vi "Rod Value Measurement.vi"() -> ()   [LabVIEW 2020]
uses:
  <vilib>/Utility/miscctls.llb/LVAnnotationListTypeDef.ctl
  <vilib>/Utility/miscctls.llb/LVStringsAndValuesArrayTypeDef_U16.ctl
  global/SettingVariable.vi
  <vilib>/Analysis/NI_AALPro.lvlib
panel:
  out "临界段周期":dbl[](array[numeric]) caption="准临界倍增周期 (s)"
  out "临界段反应性拟合值":dbl[](array[numeric]) caption="拟合反应性 (pcm)"
  out "终端反应性均值":dbl[](array[numeric]) caption="实时反应性 (pcm)"
  out "临界段反应性均值":dbl[](array[numeric]) caption="实时反应性 (pcm)"
  out "采样间隔":dbl
  out "开始时间":timestamp
  in  "打开文件":bool
  out "历史波形图":cluster{dbl, dbl, dbl[][]}(graph)
  out "终端段点数":i32 caption="终端段点数："
  out "动态段点数":i32 caption="动态段点数："
  out "左选标时刻":timestamp caption="左选标时刻：" format="%<%.2X %x>T"
  out "临界段点数":i32 caption="临界段点数："
  out "反应性记录表":string[][](table)
  in  "刻棒选择":u16(ring) caption="刻棒选择："
  in  "棒位偏移":dbl(slide) caption="棒位偏移：" min=-0.1 max=0.1 step=0.001 scale=-0.1..0.1 scale format="%#.3g"
  in  "保存表格":bool
  in  "添加记录":bool
  in  "选项卡控件":enum32{"动态段数据", "动态段曲线"}(tab)
  out "棒价值表":string[][](table) caption="动态段"
  in  "另存数据":bool
  out "价值曲线":cluster{dbl[], dbl[]}[](graph) caption="（X和Y数组）多曲线"
  out "提示信息":string="打开文件后，拖动波形图中的游标选取临界段、动态段和终端段数据进行计算。"
  out "文件信息":string
  # "临界段计算结果"
  # "终端段计算结果"
  # "坐标轴与图例"
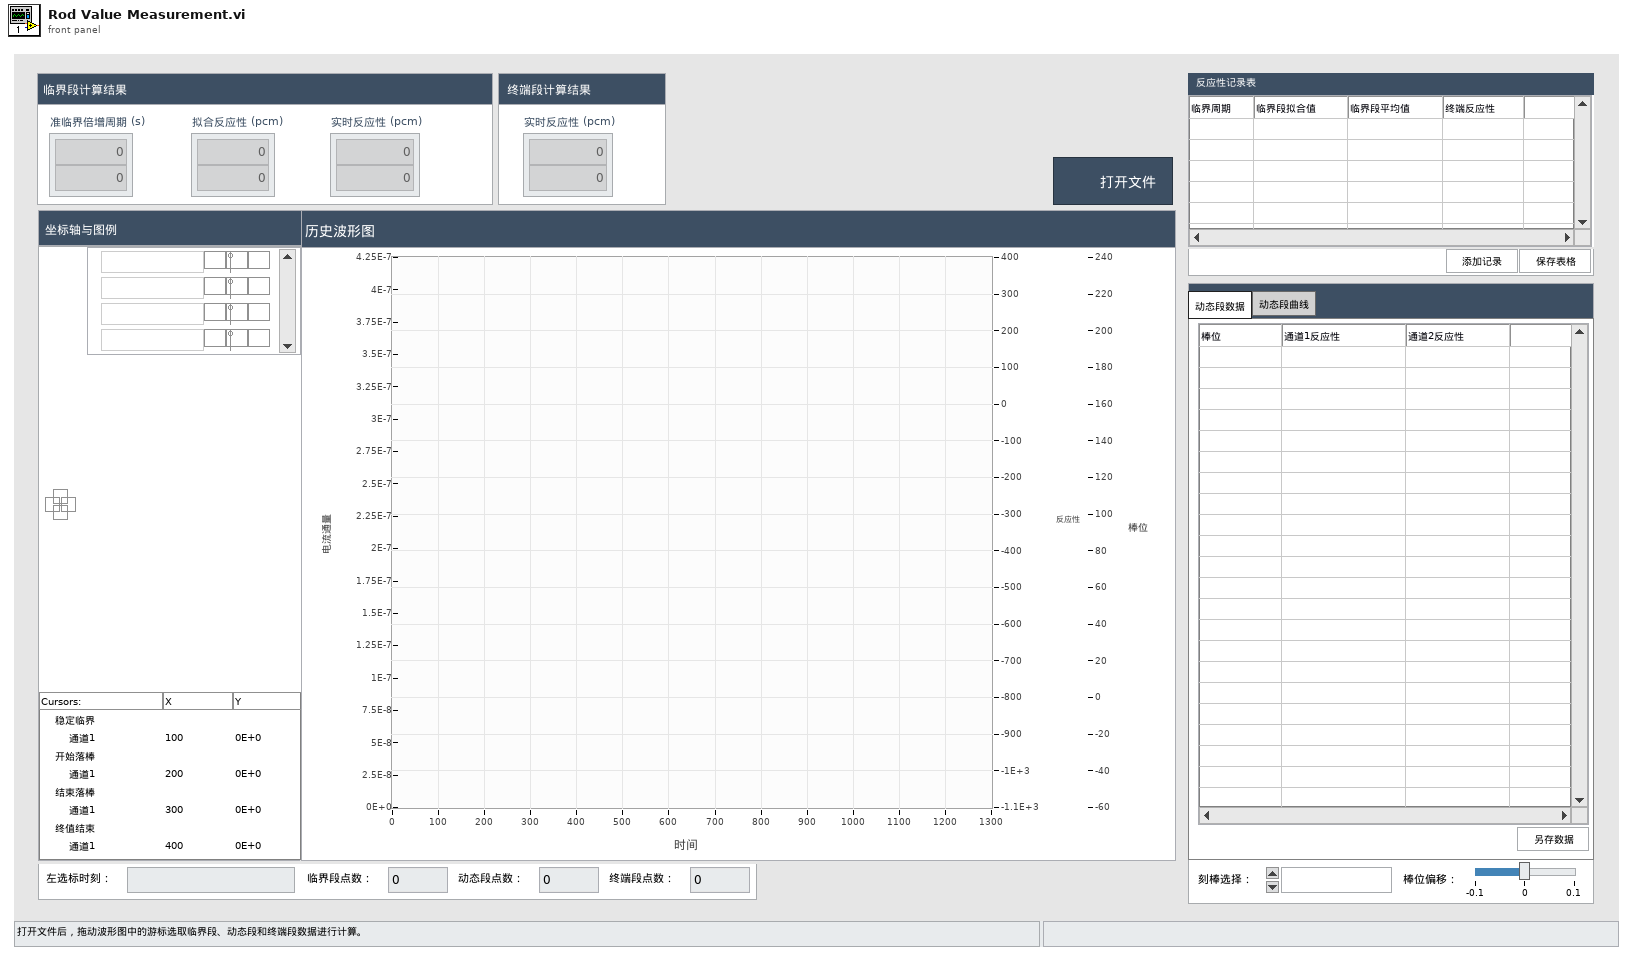
[diagram p1: front panel]
types:
  T1 = typedef "LVAnnotationListTypeDef.ctl" = cluster{"Name":string, "Color":u32, "Style":u8, "Point Style":u8, "Name Visible":bool, "Allow Drag":bool, "Annotation Mode":u32, "Plot":i32, "Index":i32, "Position":cluster{"X":dbl, "Y":dbl}, "X Scale":u32, "Y Scale":u32, "Show Arrow":bool, "Lock Name":bool, "Plot Area":i32, "Label Offset":cluster{"X":dbl, "Y":dbl}}[]
  T2 = typedef "LVStringsAndValuesArrayTypeDef_U16.ctl" = cluster{"String":string, "Value":u16}[]
  T3 = cluster{"Name":string, "Color":u32, "Style":u8, "Point Style":u8, "Name Visible":bool, "Allow Drag":bool, "Annotation Mode":u32, "Plot":i32, "Index":i32, "Position":cluster{"X":dbl, "Y":dbl}, "X Scale":u32, "Y Scale":u32, "Show Arrow":bool, "Lock Name":bool, "Plot Area":i32, "Label Offset":cluster{"X":dbl, "Y":dbl}}
  T4 = cluster{"amp min":dbl, "amp max":dbl, "damping min":dbl, "damping max":dbl, "offset min":dbl, "offset max":dbl}
  T5 = enum16{"open", "replace", "create", "open or create", "replace or create", "replace or create with confirmation"}
  T6 = typedef "LVCursorListTypeDef.ctl" = cluster{"Name":string, "Color":u32, "Style":u8, "Point Style":u8, "Name Visible":bool, "Allow Drag":bool, "Cursor Mode":u32, "Plot":i32, "Index":i32, "Position":cluster{"X":dbl, "Y":dbl}, "X Scale":u32, "Y Scale":u32, "Watch Plots":i32[], "Watch All Plots":bool, "Plot Area":i32, "Label Offset":cluster{"X":dbl, "Y":dbl}}[]
  T7 = cluster{"Name":string, "Color":u32, "Style":u8, "Point Style":u8, "Name Visible":bool, "Allow Drag":bool, "Cursor Mode":u32, "Plot":i32, "Index":i32, "Position":cluster{"X":dbl, "Y":dbl}, "X Scale":u32, "Y Scale":u32, "Watch Plots":i32[], "Watch All Plots":bool, "Plot Area":i32, "Label Offset":cluster{"X":dbl, "Y":dbl}}
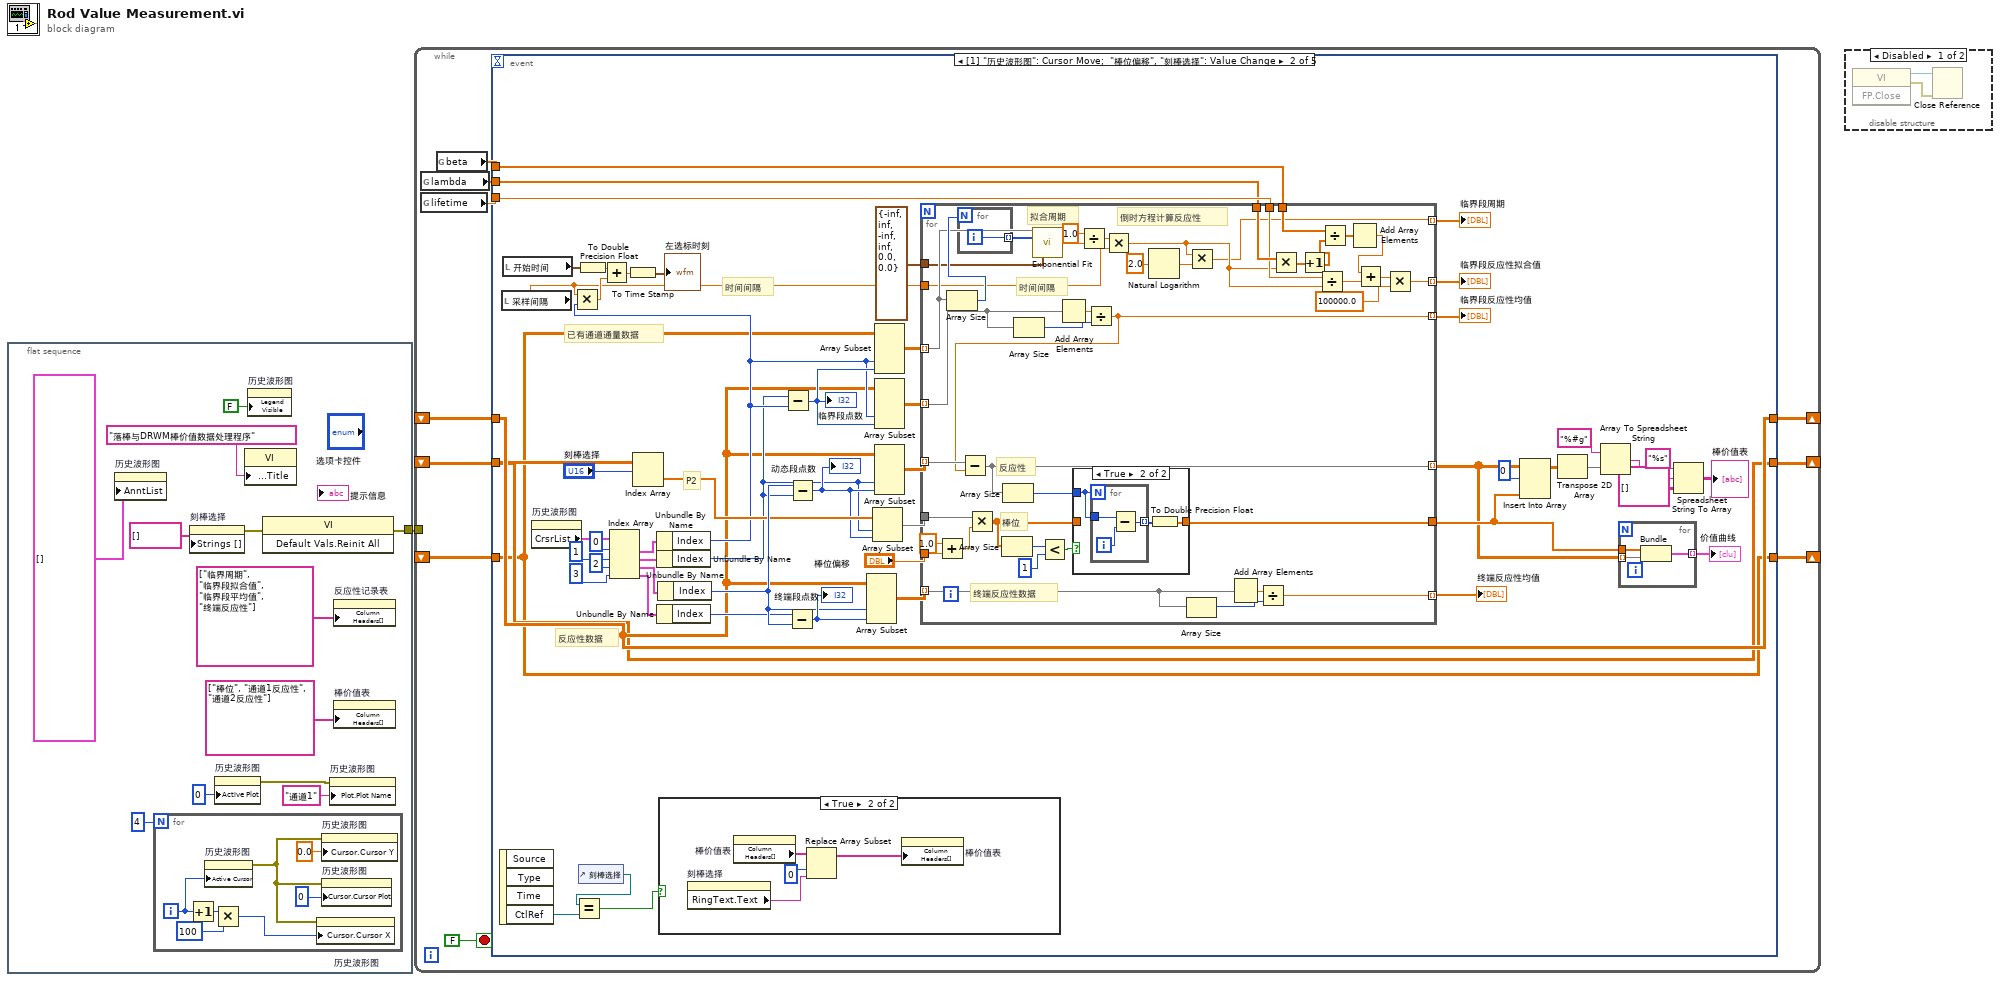
[diagram p0: block diagram]
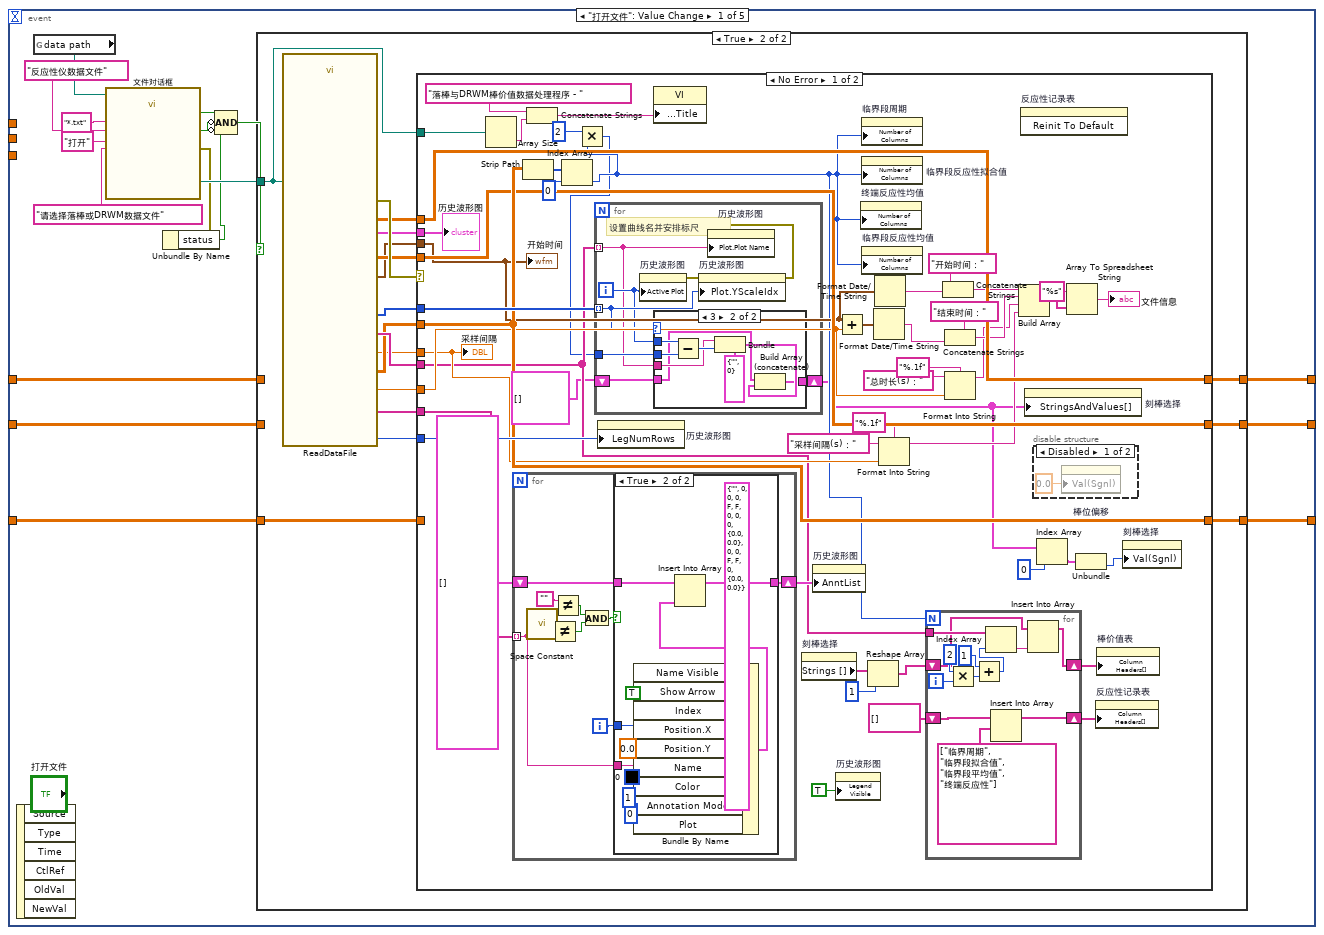
[diagram p2: hidden frame]
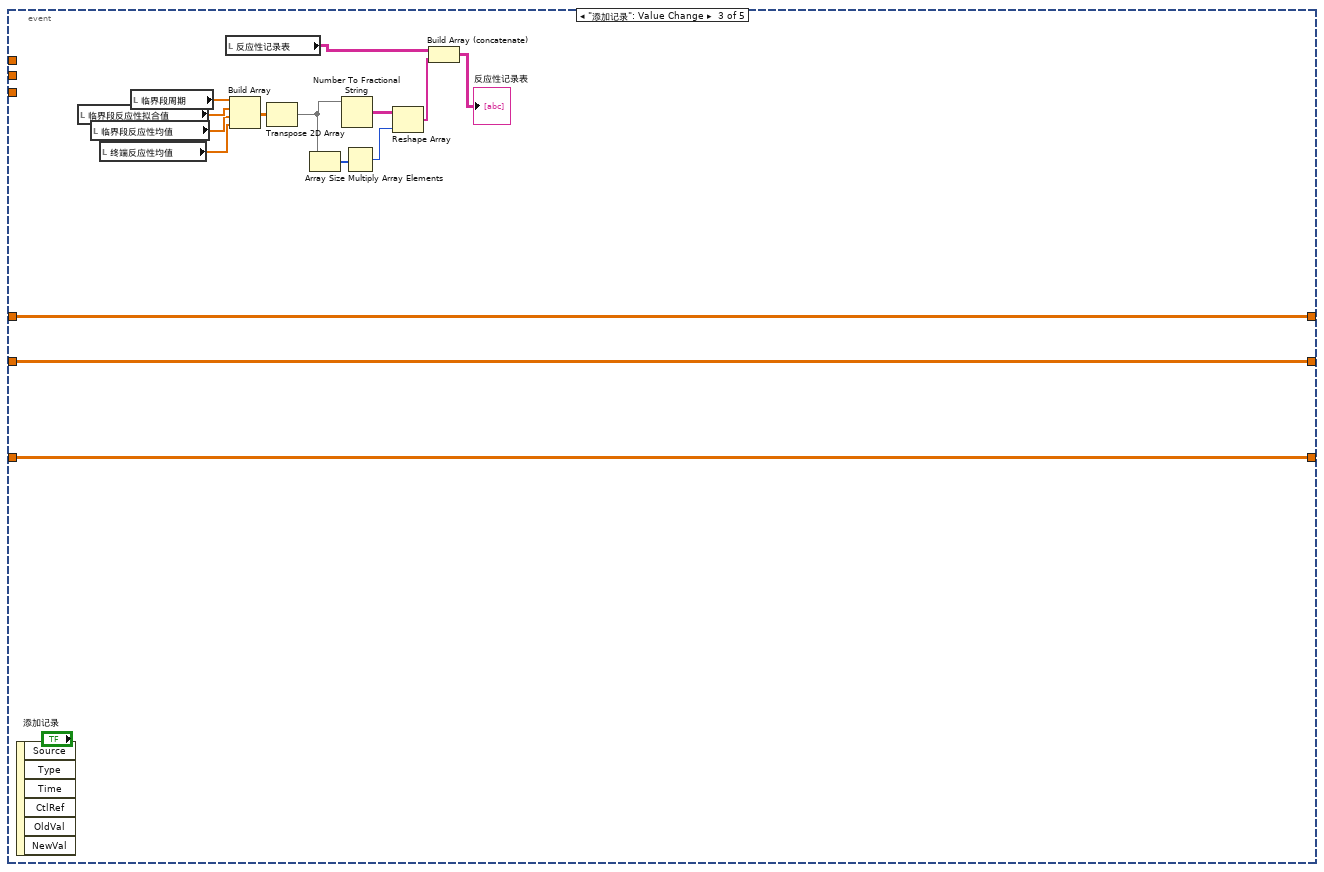
[diagram p10: hidden frame]
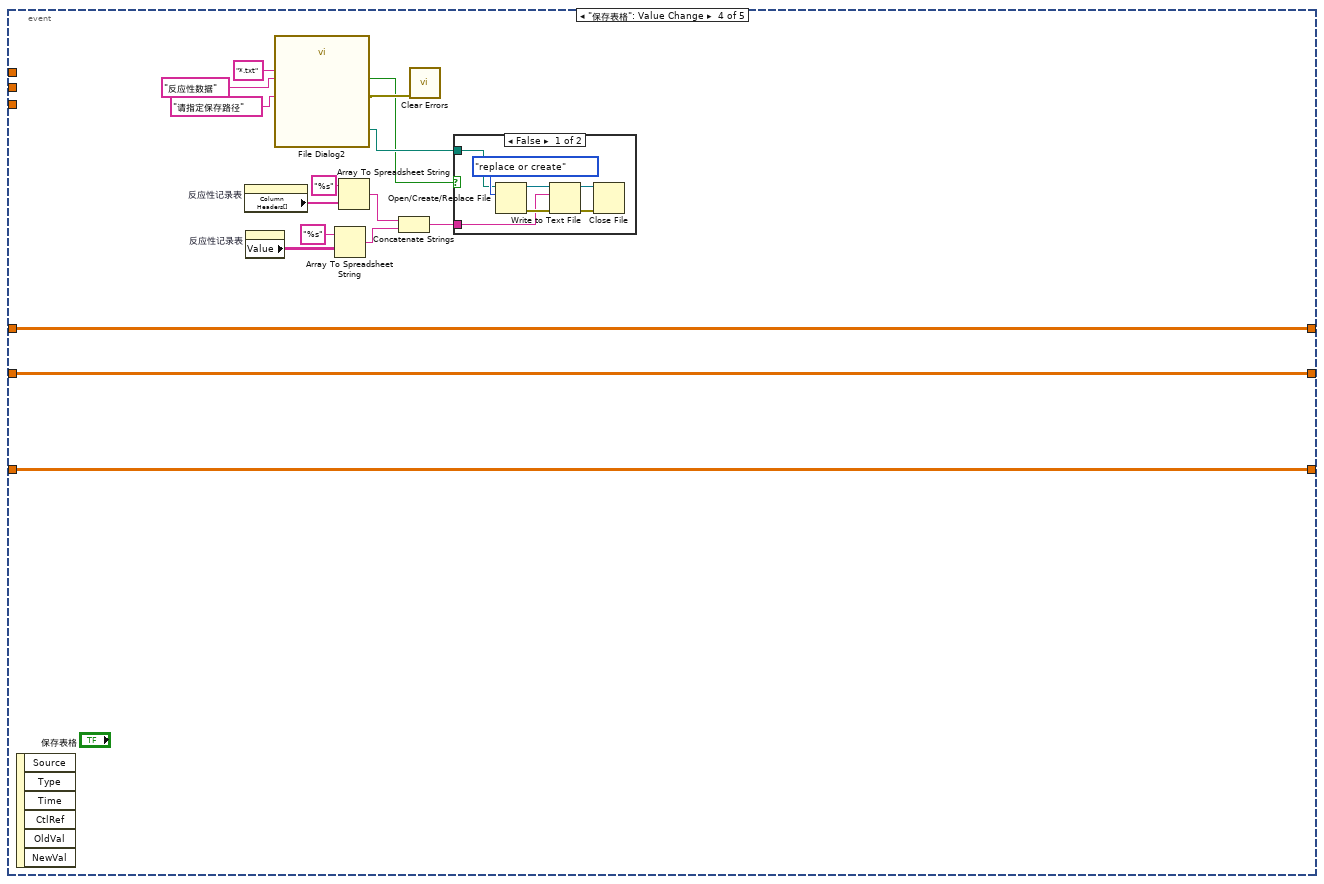
[diagram p11: hidden frame]
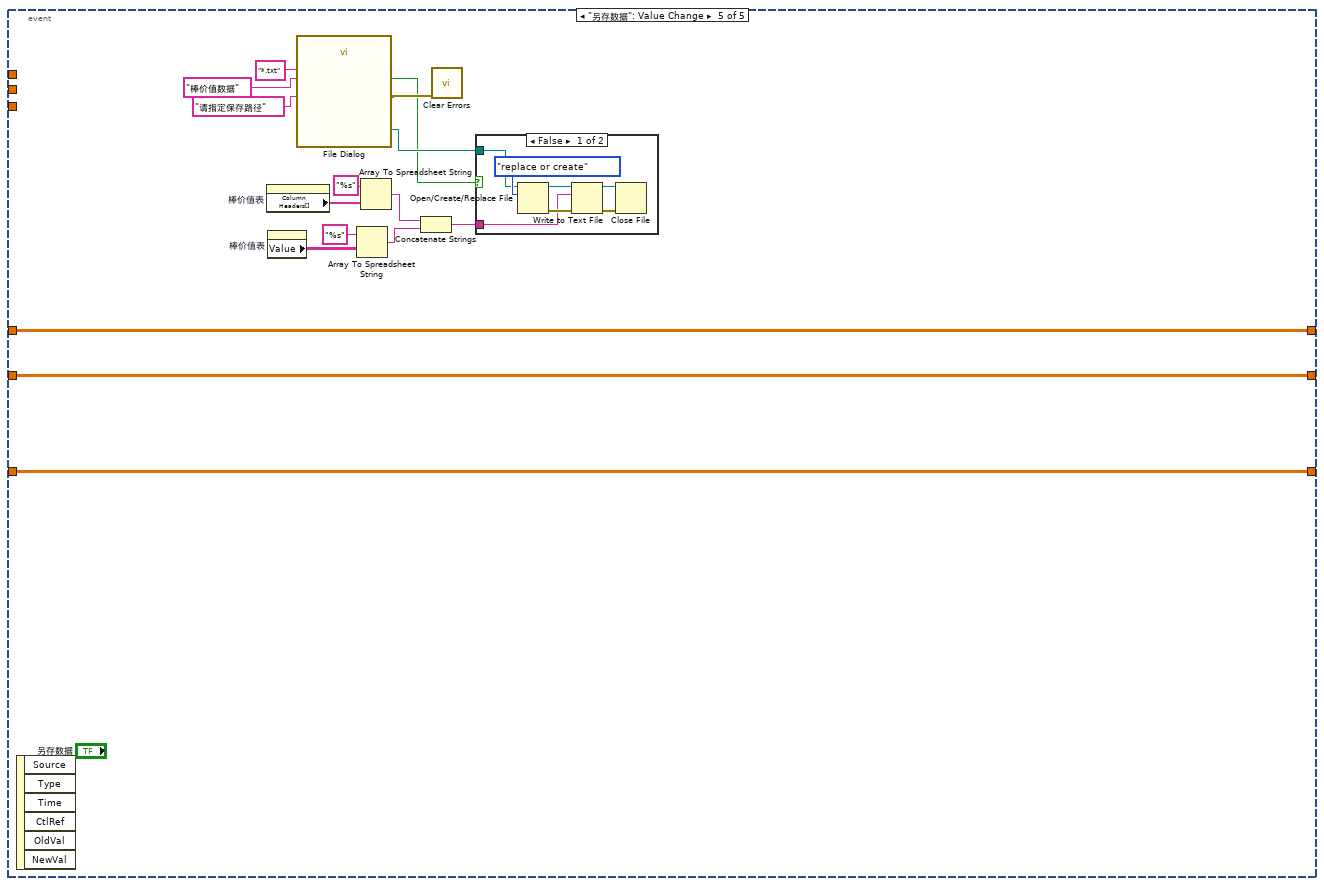
[diagram p13: hidden frame]
diagram:
  n1 = flat-sequence {
    tunnel: [w6] -> w1
    frame #0 {
      n2 = property on="历史波形图" class="WFGraph (strict)"("AnntList"=T1 [] ("Annotation List")) -> ()  [unwired: 2 in, 2 out]
      n3 = for {
        N: 4 -> [_]
        i -> [w18]
        n4 = Increment(x=w18) -> (x+1=w17:i32)
        n5 = property on="历史波形图" class="WFGraph (strict)"("Active Cursor"=w18) -> (error out=w14:errorcluster)  [unwired: 2 in, 1 out]
        n6 = Multiply(x=w17, y=100) -> (x*y=w15:i32)
        n7 = property on="历史波形图" class="WFGraph (strict)"(error in=w14, "Cursor.Cursor X"=w15) -> ()  [unwired: 1 in, 2 out]
        n8 = property on="历史波形图" class="WFGraph (strict)"(error in=w14, "Cursor.Cursor Y"=0.0 ("Cursor.Cursor Position:Cursor Y")) -> ()  [unwired: 1 in, 2 out]
        n9 = property on="历史波形图" class="WFGraph (strict)"(error in=w14, "Cursor.Cursor Plot"=0 ("Cursor.Cursor Index")) -> ()  [unwired: 1 in, 2 out]
      }
      n10 = property on="刻棒选择" class="Ring (strict)"("Strings []"=string[] []) -> (error out=w5:errorcluster)  [unwired: 2 in, 1 out]
      n11 = property on="历史波形图" class="WFGraph (strict)"("Active Plot"=u32 0) -> (error out=w9:errorcluster)  [unwired: 2 in, 1 out]
      n12 = property class="VI"("Front Panel.Title"="落棒与DRWM棒价值数据处理程序" ("Front Panel Window:Title")) -> ()  [unwired: 2 in, 2 out]
      n13 = property on="历史波形图" class="WFGraph (strict)"("Legend Visible"=FALSE ("Legend:Visible")) -> ()  [unwired: 2 in, 2 out]
      n14 = invoke class="VI" method="Default Vals.Reinit All"(error in=w5) -> (error out=w6:errorcluster)  [unwired: 2 in, 2 out]
      n15 = property on="历史波形图" class="WFGraph (strict)"(error in=w9, "Plot.Plot Name"="通道1") -> ()  [unwired: 1 in, 2 out]
      n16 = property on="反应性记录表" class="Tbl (strict)"("Column Headers[]"=string[] ["临界周期", "临界段拟合值", "临界段平均值", "终端反应性"] ("行首字符串[]")) -> ()  [unwired: 2 in, 2 out]
      n17 = property on="棒价值表" class="Tbl (strict)"("Column Headers[]"=string[] ["棒位", "通道1反应性", "通道2反应性"] ("添加的数组")) -> ()  [unwired: 2 in, 2 out]
    }
  }
  n18 = while {
    shift-right: [w29] -> _
    shift-left: _ -> [w28]
    shift-right: [w27] -> _
    shift-left: _ -> [w25]
    shift-right: [w26] -> _
    shift-left: _ -> [w24]
    tunnel: w1 -> [_]
    stop <- FALSE stop-if-true
    n19 = global read "SettingVariable.vi" "lambda"() -> (w22:dbl[])
    n20 = global read "SettingVariable.vi" "lifetime"() -> (w21:dbl)
    n21 = global read "SettingVariable.vi" "beta"() -> (w23:dbl[])
    n22 = event shown="[1] \"历史波形图\": Cursor Move;  \"棒位偏移\", \"刻棒选择\": Value Change" {
      selector: _ -> [_ _ _ _ _]
      dyn-events: _ -> [_ _ _ _ _]
      timeout: _ -> [_ _ _ _ _]
      tunnel: [w42 w178 w297 w313 w332] -> w29
      tunnel: w28 -> [w41 w178 w297 w313 w332]
      tunnel: [w40 w180 w299 w315 w334] -> w27
      tunnel: [w39 w179 w298 w314 w333] -> w26
      tunnel: w25 -> [w38 w180 w299 w315 w334]
      tunnel: w24 -> [w37 w179 w298 w314 w333]
      tunnel: w23 -> [_ w226 _ _ _]
      tunnel: w21 -> [_ w225 _ _ _]
      tunnel: w22 -> [_ w224 _ _ _]
      event "打开文件": Value Change {
        n23 = event-data() -> ()  [unwired: 1 in, 6 out]
        n24 = global read "SettingVariable.vi" "data path"() -> (w31:path)
        n25 = call "文件对话框"("start path"=w31, "prompt"="请选择落棒或DRWM数据文件", "button label"="打开", "pattern (all files)"="*.txt", "pattern label"="反应性仪数据文件") -> ("selected path"=w47:path, "exists"=w35:bool, "cancelled"=w34:bool, "error out"=w36:errorcluster)  [unwired: 7 in]
        n26 = Unbundle By Name(w36) -> ("status"=w33:bool)
        n27 = Compound Arithmetic op=AND(w35, invert w34, invert w33) -> (w32:bool)
        n28 = case shown="True" w32 {
          tunnel: w47 -> [_ w51]
          tunnel: [w50 w59] -> w42
          tunnel: w41 -> [w50 w58]
          tunnel: [w49 w55] -> w40
          tunnel: [w48 w54] -> w39
          tunnel: w38 -> [w49 _]
          tunnel: w37 -> [w48 _]
          frame False {
          }
          frame True {
            n29 = call "ReadDataFile.vi"("file path (dialog if empty)"=w51) -> ("曲线对应标尺编号"=w62:i32[], "曲线名"=w61:string[], "通量数据"=w60:dbl[][], "时间间隔"=w57:dbl, "P2数据"=w53:dbl[][], "曲线数"=w64:i32, "开始时间"=w52:timestamp, "反应性数据"=w56:dbl[][], "总时长(s)"=w65:dbl, "error out"=w67:errorcluster, "备注数组"=w63:string[], "波形簇"=w66:cluster{dbl, dbl, dbl[][]})  [unwired: 2 in, 1 out]
            n30 = case shown="No Error" w67 {
              tunnel: w66 -> [w117 _]
              tunnel: w65 -> [w97 _]
              tunnel: w64 -> [w116 _]
              tunnel: w63 -> [w113 _]
              tunnel: w62 -> [w112 _]
              tunnel: w61 -> [w84 _]
              tunnel: w60 -> [w109 _]
              tunnel: [w109 w171] -> w59
              tunnel: w58 -> [_ w171]
              tunnel: w57 -> [w95 _]
              tunnel: w56 -> [w108 w170]
              tunnel: [w108 w170] -> w55
              tunnel: [w107 w169] -> w54
              tunnel: w53 -> [w107 w169]
              tunnel: w52 -> [w102 _]
              tunnel: w51 -> [w70 _]
              frame No Error {
                n31 = Strip Path(path=w70) -> (name=w71:string)  [unwired: 1 out]
                n32 = for {
                  tunnel: w113 -> [w151] mode=indexing
                  shift-right: [w153] -> w115
                  shift-left: T1 [] ("注释列表") -> [w154]
                  i -> [w155]
                  n33 = call <vilib>:"Space Constant.vi"() -> ("String"=w156:string)
                  n34 = Not Equal?(x=w156, y=w151) -> (x != y?=w149:bool)
                  n35 = Not Equal?(x="", y=w151) -> (x != y?=w150:bool)
                  n36 = And(x=w150, y=w149) -> (x .and. y?=w148:bool)
                  n37 = case shown="True" w148 {
                    tunnel: w151 -> [_ w163]
                    tunnel: w155 -> [_ w165]
                    tunnel: w154 -> [w157 w168]
                    tunnel: [w157 w167] -> w153
                    frame False {
                    }
                    frame True {
                      w166 = TRUE ("Show Arrow")
                      n38 = Bundle By Name(cluster=T3 {"Name"="", "Color"=0, "Style"=0, "Point Style"=0, "Name Visible"=FALSE, "Allow Drag"=FALSE, "Annotation Mode"=0, "Plot"=0, "Index"=0, "Position"={"X"=0.0, "Y"=0.0}, "X Scale"=0, "Y Scale"=0, "Show Arrow"=FALSE, "Lock Name"=FALSE, "Plot Area"=0, "Label Offset"={"X"=0.0, "Y"=0.0}} ("元素"), "Name Visible"=w166, "Show Arrow"=w166, "Index"=w165, "Position.X"=w165, "Position.Y"=0.0 ("Y"), "Name"=w163, "Color"=u32 0, "Annotation Mode"=u32 1, "Plot"=0) -> (w164:T3)
                      n39 = Insert Into Array(array=w168, new element=w164) -> (w167:T1)  [unwired: 1 in]
                    }
                  }
                }
                n40 = Array Size(array=w109) -> (size(s)=w111:i32[])
                n41 = Concatenate Strings("落棒与DRWM棒价值数据处理程序 - " ("string"), w71) -> (w72:string)
                n42 = Index Array(array=w111, index=0 ("索引")) -> (element=w83:i32)
                n43 = Multiply(x=2, y=w83) -> (x*y=w81:i32)
                n44 = for {
                  tunnel: w112 -> [w136] mode=indexing
                  tunnel: w84 -> [w133] mode=indexing
                  tunnel: w81 -> [w134]
                  shift-right: [w131] -> w68
                  shift-left: T2 [] ("Strings And Values []") -> [w132]
                  i -> [w135]
                  # "设置曲线名并安排标尺"
                  n45 = property on="历史波形图" class="WFGraph (strict)"("Active Plot"=w135) -> (error out=w138:errorcluster)  [unwired: 2 in, 1 out]
                  n46 = case shown="3" w136 {
                    tunnel: w135 -> [_ w146]
                    tunnel: w134 -> [_ w147]
                    tunnel: w133 -> [_ w144]
                    tunnel: w132 -> [w139 w142]
                    tunnel: [w139 w140] -> w131
                    frame 0, Default {
                    }
                    frame 3 {
                      n47 = Subtract(x=w146, y=w147) -> (x-y=w145:i32)
                      n48 = Bundle(cluster=cluster{"String":string, "Value":u16} {"String"="", "Value"=0}, "String"=w144, "Value"=w145) -> (w141:cluster{"String":string, "Value":u16})
                      n49 = Build Array (concatenate)(w142, w141) -> (w140:T2)
                    }
                  }
                  n50 = property on="历史波形图" class="WFGraph (strict)"(error in=w138, "Plot.YScaleIdx"=w136) -> (error out=w137:errorcluster)  [unwired: 1 in, 1 out]
                  n51 = property on="历史波形图" class="WFGraph (strict)"(error in=w137, "Plot.Plot Name"=w133) -> ()  [unwired: 1 in, 2 out]
                }
                n52 = property on="历史波形图" class="WFGraph (strict)"("LegNumRows"=w116) -> ()  [unwired: 2 in, 2 out]
                n53 = property class="VI"("Front Panel.Title"=w72) -> ()  [unwired: 2 in, 2 out]
                n54 = property on="刻棒选择" class="Ring (strict)"() -> ("Strings []"=w79:string[])  [unwired: 2 in, 2 out]
                n55 = property on="历史波形图" class="WFGraph (strict)"("AnntList"=w115) -> ()  [unwired: 2 in, 2 out]
                n56 = property on="历史波形图" class="WFGraph (strict)"("Legend Visible"=TRUE ("Legend:Visible")) -> ()  [unwired: 2 in, 2 out]
                n57 = Add(x=w102, y=w97) -> (x+y=w103:timestamp)
                n58 = property on="终端反应性均值" class="Arr (strict)"("Number of Columns"=w83) -> ()  [unwired: 2 in, 2 out]
                n59 = property on="临界段周期" class="Arr (strict)"("Number of Columns"=w83) -> ()  [unwired: 2 in, 2 out]
                n60 = property on="临界段反应性拟合值" class="Arr (strict)"("Number of Columns"=w83) -> ()  [unwired: 2 in, 2 out]
                n61 = property on="临界段反应性均值" class="Arr (strict)"("Number of Columns"=w83) -> ()  [unwired: 2 in, 2 out]
                n62 = Reshape Array(w79, 1 ("dimension size")) -> (w77:string[])
                n63 = Format Date/Time String(seconds (now)=w103) -> (date/time string=w98:string)  [unwired: 2 in]
                n64 = Format Date/Time String(seconds (now)=w102) -> (date/time string=w100:string)  [unwired: 2 in]
                n65 = Format Into String(format string="%.1f", initial string="采样间隔(s)：", w95) -> (resulting string=w88:string)  [unwired: 1 in, 1 out]
                n66 = for {
                  N: w83 -> [_]
                  tunnel: w84 -> [w128]
                  shift-right: [w123] -> w106
                  shift-left: w77 -> [w122]
                  shift-right: [w119] -> w104
                  shift-left: string[] [] ("行首字符串[]") -> [w120]
                  i -> [w130]
                  n67 = Multiply(x=2, y=w130) -> (x*y=w127:i32)
                  n68 = Add(x=1, y=w127) -> (x+y=w125:i32)
                  n69 = Index Array(array=w128, index=w125) -> (element=w124:string)
                  n70 = Insert Into Array(array=w120, new element=string[] ["临界周期", "临界段拟合值", "临界段平均值", "终端反应性"] ("行首字符串[]")) -> (w119:string[])  [unwired: 1 in]
                  n71 = Insert Into Array(array=w122, new element=w124) -> (w123:string[])  [unwired: 1 in]
                }
                n72 = Concatenate Strings("开始时间：" ("string"), w100) -> (w93:string)
                n73 = Concatenate Strings("结束时间：" ("string"), w98) -> (w90:string)
                n74 = Format Into String(format string="%.1f", initial string="总时长(s)：", w97) -> (resulting string=w89:string)  [unwired: 1 in, 1 out]
                n75 = Build Array(w93, w90, w89, w88) -> (w92:string[])
                n76 = invoke on="反应性记录表" class="Tbl (strict)" method="Reinit To Default"() -> ()  [unwired: 3 in, 3 out]
                n77 = property on="刻棒选择" class="Ring (strict)"("StringsAndValues[]"=w68) -> ()  [unwired: 2 in, 2 out]
                n78 = disable-structure shown="Disabled" {
                  frame Disabled {
                    n79 = property on="棒位偏移" class="Slide (strict)"("Val(Sgnl)"=0.0 ("Value (Signaling)")) -> ()  [unwired: 2 in, 2 out]
                  }
                  frame Enabled {
                  }
                }
                n80 = Index Array(array=w68, index=0) -> (element=w75:cluster{"String":string, "Value":u16})
                n81 = Array To Spreadsheet String(array=w92, 3:"%s" ("format string")) -> (spreadsheet string=→"文件信息":string)  [unwired: 1 in]
                n82 = Unbundle(w75) -> ("Value"=w74:u16)  [unwired: 1 out]
                n83 = property on="反应性记录表" class="Tbl (strict)"("Column Headers[]"=w104) -> ()  [unwired: 2 in, 2 out]
                n84 = property on="棒价值表" class="Tbl (strict)"("Column Headers[]"=w106) -> ()  [unwired: 2 in, 2 out]
                n85 = property on="刻棒选择" class="Ring (strict)"("Val(Sgnl)"=w74) -> ()  [unwired: 2 in, 2 out]
                "历史波形图" <- w117
                "开始时间" <- w102
                "采样间隔" <- w95
              }
              frame Error {
              }
            }
          }
        }
      }
      event "历史波形图": Cursor Move; "棒位偏移", "刻棒选择": Value Change {
        # "反应性数据"
        # "P2"
        # "时间间隔"
        # "已有通道通量数据"
        n86 = event-data() -> ("CtlRef"=w173:refnum<vi>)  [unwired: 1 in, 3 out]
        n87 = local read "采样间隔"() -> (w176:dbl)
        n88 = local read "开始时间"() -> (w177:timestamp)
        n89 = property on="历史波形图" class="WFGraph (strict)"() -> ("CrsrList"=w219:T6)  [unwired: 2 in, 2 out]
        n90 = To Double Precision Float(number=w177) -> (double precision float=w211:dbl)
        n91 = control-ref of="刻棒选择"() -> (w174:refnum<vi>)
        n92 = Equal?(x=w174, y=w173) -> (x = y?=w172:bool)
        n93 = Index Array(array=w219, index #1=0 ("index"), index #2=1 ("index"), index #3=2 ("索引"), index #4=3 ("索引")) -> (element #1=w221:T7, element #2=w223:T7, element #3=w204:T7, element #4=w203:T7)
        n94 = Index Array(array=w179, index (row)="刻棒选择") -> (element=w192:dbl[])  [unwired: 1 in]
        n95 = Unbundle By Name(w221) -> ("Index"=w183:i32)
        n96 = Multiply(x=w176, y=w183) -> (x*y=w208:dbl)
        n97 = Add(x=w211, y=w208) -> (x+y=w210:dbl)
        n98 = To Time Stamp(1:w210) -> (0:→"左选标时刻":timestamp)
        n99 = Unbundle By Name(w223) -> ("Index"=w182:i32)
        n100 = Unbundle By Name(w203) -> ("Index"=w200:i32)
        n101 = Unbundle By Name(w204) -> ("Index"=w201:i32)
        n102 = case shown="True" w172 {
          frame False {
          }
          frame True {
            n103 = property on="刻棒选择" class="Ring (strict)"() -> ("RingText.Text"=w228:string)  [unwired: 2 in, 2 out]
            n104 = property on="棒价值表" class="Tbl (strict)"() -> ("Column Headers[]"=w230:string[])  [unwired: 2 in, 2 out]
            n105 = Replace Array Subset(array=w230, new element=w228, index=0) -> (w227:string[])
            n106 = property on="棒价值表" class="Tbl (strict)"("Column Headers[]"=w227) -> ()  [unwired: 2 in, 2 out]
          }
        }
        n107 = Subtract(x=w182, y=w183) -> (x-y=w216:i32)
        "临界段点数" <- w216
        n108 = Subtract(x=w200, y=w201) -> (x-y=w202:i32)
        "终端段点数" <- w202
        n109 = Subtract(x=w201, y=w182) -> (x-y=w191:i32)
        "动态段点数" <- w191
        n110 = Array Subset(array=w180, index (col)=w201, length (col)=w202) -> (w199:dbl[][])  [unwired: 2 in]
        n111 = Array Subset(array=w192, index=w182, length=w191) -> (w197:dbl[])
        n112 = Array Subset(array=w178, index (col)=w183, length (col)=w216) -> (w218:dbl[][])  [unwired: 2 in]
        n113 = Array Subset(array=w180, index (col)=w183, length (col)=w216) -> (w217:dbl[][])  [unwired: 2 in]
        n114 = Array Subset(array=w180, index (col)=w182, length (col)=w191) -> (w205:dbl[][])  [unwired: 2 in]
        n115 = for {
          tunnel: w218 -> [w261] mode=indexing
          tunnel: w225 -> [w273]
          tunnel: w226 -> [w276]
          tunnel: w224 -> [w275]
          tunnel: w217 -> [w246] mode=indexing
          tunnel: [w248] -> w214 mode=indexing
          tunnel: [w245] -> w181 mode=indexing
          tunnel: [w274] -> w215 mode=indexing
          tunnel: [w252] -> w213 mode=indexing
          tunnel: w176 -> [w254]
          tunnel: T4 {"amp min"=-inf, "amp max"=inf, "damping min"=-inf, "damping max"=inf, "offset min"=0.0, "offset max"=0.0} ("parameter bounds") -> [w256]
          tunnel: w205 -> [w247] mode=indexing
          tunnel: w199 -> [w249] mode=indexing
          tunnel: w197 -> [w244]
          tunnel: "棒位偏移" -> [w243]
          tunnel: [w236] -> w185 mode=indexing
          tunnel: [w234] -> w187
          # "棒位"
          # "反应性"
          # "终端反应性数据"
          # "时间间隔"
          # "拟合周期"
          # "倒时方程计算反应性"
          n116 = Add(x=1.0, y=w243) -> (x+y=w241:dbl)
          n117 = Array Size(array=w261) -> (size(s)=w263:i32)
          n118 = for {
            N: w263 -> [_]
            tunnel: [w284] -> w262 mode=indexing
            i -> [w284]
          }
          n119 = Multiply(x=w244, y=w241) -> (x*y=w240:dbl[])
          n120 = Array Size(array=w240) -> (size(s)=w239:i32)
          n121 = Array Size(array=w246) -> (size(s)=w264:i32)
          n122 = call <vilib>:"Exponential Fit.vi"("Y"=w261, "X"=w262, "parameter bounds"=w256) -> ("damping"=w260:dbl)  [unwired: 7 in, 5 out]
          n123 = Less?(x=w239, y=1) -> (x < y?=w237:bool)
          n124 = Add Array Elements(numeric array=w246) -> (sum=w272:dbl)
          n125 = Divide(x=1.0, y=w260) -> (x/y=w255:dbl)
          n126 = Divide(x=w272, y=w264) -> (x/y=w245:dbl)
          n127 = Subtract(x=w247, y=w245) -> (x-y=w236:dbl[])
          n128 = Array Size(array=w236) -> (size(s)=w235:i32)
          n129 = case shown="True" w237 {
            tunnel: w240 -> [w277 _]
            tunnel: w235 -> [_ w280]
            tunnel: [w277 w278] -> w234
            frame False {
            }
            frame True {
              n130 = for {
                N: w280 -> [_]
                tunnel: w280 -> [w283]
                tunnel: [w281] -> w279 mode=indexing
                i -> [w282]
                n131 = Subtract(x=w283, y=w282) -> (x-y=w281:i32)
              }
              n132 = To Double Precision Float(number=w279) -> (double precision float=w278:dbl[])
            }
          }
          n133 = Multiply(x=w255, y=w254) -> (x*y=w253:dbl)
          n134 = Natural Logarithm(1:sgl 2.0) -> (0:w257:sgl)
          n135 = Array Size(array=w249) -> (size(s)=w250:i32)
          n136 = Multiply(x=w253, y=w257) -> (x*y=w252:dbl)
          n137 = Add Array Elements(numeric array=w249) -> (sum=w251:dbl)
          n138 = Divide(x=w251, y=w250) -> (x/y=w248:dbl)
          n139 = Multiply(x=w275, y=w253) -> (x*y=w265:dbl[])
          n140 = Increment(x=w265) -> (x+1=w266:dbl[])
          n141 = Divide(x=w273, y=w253) -> (x/y=w269:dbl)
          n142 = Divide(x=w276, y=w266) -> (x/y=w271:dbl[])
          n143 = Add Array Elements(numeric array=w271) -> (sum=w270:dbl)
          n144 = Add(x=w270, y=w269) -> (x+y=w268:dbl)
          n145 = Multiply(x=w268, y=sgl 100000.0) -> (x*y=w274:dbl)
        }
        "临界段反应性均值" <- w181
        "终端反应性均值" <- w214
        "临界段反应性拟合值" <- w215
        "临界段周期" <- w213
        n146 = Insert Into Array(array=w185, index (row)=0 ("索引 (行)"), new element=w187) -> (w190:dbl[][])  [unwired: 1 in]
        n147 = Transpose 2D Array(2D array=w190) -> (transposed array=w189:dbl[][])
        n148 = Array To Spreadsheet String(array=w189, 3:"%#g" ("格式字符串")) -> (spreadsheet string=w184:string)  [unwired: 1 in]
        n149 = for {
          tunnel: w187 -> [w231]
          tunnel: w185 -> [w232] mode=indexing
          tunnel: [w233] -> w186 mode=indexing
          n150 = Bundle "Bundle"(w231, w232) -> (w233:cluster{dbl[], dbl[]})  [unwired: 1 in]
        }
        "价值曲线" <- w186
        n151 = Spreadsheet String To Array(format string="%s" ("格式字符串"), spreadsheet string=w184, array type (2D Dbl)=string[][] [] ("添加的数组")) -> (array=→"棒价值表":string[][])  [unwired: 1 in]
      }
      event "添加记录": Value Change {
        n152 = event-data() -> ()  [unwired: 1 in, 6 out]
        n153 = local read "临界段反应性拟合值"() -> (w295:dbl[])
        n154 = local read "临界段反应性均值"() -> (w294:dbl[])
        n155 = local read "终端反应性均值"() -> (w293:dbl[])
        n156 = local read "临界段周期"() -> (w296:dbl[])
        n157 = local read "反应性记录表"() -> (w291:string[][])
        n158 = Build Array(w296, w295, w294, w293) -> (w285:dbl[][])
        n159 = Transpose 2D Array(2D array=w285) -> (transposed array=w286:dbl[][])
        n160 = Array Size(array=w286) -> (size(s)=w288:i32[])
        n161 = Number To Fractional String(number=w286) -> (F-format string=w292:string[][])  [unwired: 3 in]
        n162 = Multiply Array Elements(1:w288) -> (0:w287:i32)
        n163 = Reshape Array(w292, w287) -> (w290:string[])
        n164 = Build Array (concatenate)(w291, w290) -> (→"反应性记录表":string[][])
      }
      event "保存表格": Value Change {
        n165 = event-data() -> ()  [unwired: 1 in, 6 out]
        n166 = property on="反应性记录表" class="Tbl (strict)"() -> ("Column Headers[]"=w312:string[])  [unwired: 2 in, 2 out]
        n167 = property on="反应性记录表" class="Tbl (strict)"() -> ("Value"=w309:string[][])  [unwired: 2 in, 2 out]
        n168 = call "File Dialog2"("prompt"="请指定保存路径" ("提示"), "pattern (all files)"="*.txt" ("类型（所有文件）"), "pattern label"="反应性数据" ("默认名称")) -> ("selected path"=w306:path, "cancelled"=w305:bool, "error out"=w307:errorcluster)  [unwired: 9 in, 1 out]
        n169 = Array To Spreadsheet String(array=w309, 3:"%s" ("format string")) -> (spreadsheet string=w308:string)  [unwired: 1 in]
        n170 = Array To Spreadsheet String(array=w312, 3:"%s" ("格式字符串")) -> (spreadsheet string=w311:string)  [unwired: 1 in]
        n171 = Concatenate Strings(w311, w308) -> (w310:string)
        n172 = call <vilib>:"Clear Errors.vi"("error in (no error)"=w307) -> ()  [unwired: 5 in, 2 out]
        n173 = case shown="False" w305 {
          tunnel: w310 -> [w317 _]
          tunnel: w306 -> [w316 _]
          frame False {
            n174 = Open/Create/Replace File(file path (use dialog)=w316, operation (0:open)=T5."replace or create") -> (refnum out=w320:refnum<file>, error out=w322:errorcluster)  [unwired: 4 in, 1 out]
            n175 = Write to Text File(file (use dialog)=w320, text=w317, error in=w322) -> (refnum out=w319:refnum<file>, error out=w318:errorcluster)  [unwired: 1 in, 1 out]
            n176 = Close File(refnum=w319, error in=w318) -> ()  [unwired: 2 out]
          }
          frame True {
          }
        }
      }
      event "另存数据": Value Change {
        n177 = event-data() -> ()  [unwired: 1 in, 6 out]
        n178 = property on="棒价值表" class="Tbl (strict)"() -> ("Column Headers[]"=w338:string[])  [unwired: 2 in, 2 out]
        n179 = property on="棒价值表" class="Tbl (strict)"() -> ("Value"=w331:string[][])  [unwired: 2 in, 2 out]
        n180 = call "File Dialog"("prompt"="请指定保存路径" ("提示"), "pattern (all files)"="*.txt" ("类型（所有文件）"), "pattern label"="棒价值数据" ("默认名称")) -> ("selected path"=w327:path, "cancelled"=w326:bool, "error out"=w328:errorcluster)  [unwired: 9 in, 1 out]
        n181 = Array To Spreadsheet String(array=w331, 3:"%s" ("format string")) -> (spreadsheet string=w330:string)  [unwired: 1 in]
        n182 = Array To Spreadsheet String(array=w338, 3:"%s" ("格式字符串")) -> (spreadsheet string=w336:string)  [unwired: 1 in]
        n183 = Concatenate Strings(w336, w330) -> (w335:string)
        n184 = call <vilib>:"Clear Errors.vi"("error in (no error)"=w328) -> ()  [unwired: 5 in, 2 out]
        n185 = case shown="False" w326 {
          tunnel: w335 -> [w340 _]
          tunnel: w327 -> [w339 _]
          frame False {
            n186 = Open/Create/Replace File(file path (use dialog)=w339, operation (0:open)=T5."replace or create") -> (refnum out=w343:refnum<file>, error out=w345:errorcluster)  [unwired: 4 in, 1 out]
            n187 = Write to Text File(file (use dialog)=w343, text=w340, error in=w345) -> (refnum out=w342:refnum<file>, error out=w341:errorcluster)  [unwired: 1 in, 1 out]
            n188 = Close File(refnum=w342, error in=w341) -> ()  [unwired: 2 out]
          }
          frame True {
          }
        }
      }
    }
  }
  n189 = disable-structure shown="Disabled" {
    frame Disabled {
      n190 = invoke class="VI" method="FP.Close"() -> (reference out=w347:refnum<vi>, error out=w346:errorcluster)  [unwired: 3 in, 1 out]
      n191 = Close Reference(reference=w347, error in (no error)=w346) -> ()  [unwired: 1 out]
    }
    frame Enabled {
    }
  }
